vi "Lab1-my.vi"() -> ()   [LabVIEW 2013]
uses:
  <vilib>/Instr/_visa.llb/VISA Configure Serial Port (Instr).vi
panel:
  in  "file (use dialog)":path
  in  "stop everything":bool
  in  "send request":bool
  in  "Timeout [ms]":u32=5000
  out "answer":string
  in  "request":string
  in  "parity (0:none)":enum16{"None", "Odd", "Even", "Mark", "Space"}(ring)
  in  "data bits (8)":u16=8 min=5 max=8 step=1
  in  "baud rate (9600)":u32=9600
  in  "VISA resource name":refnum<visa-resource-name>
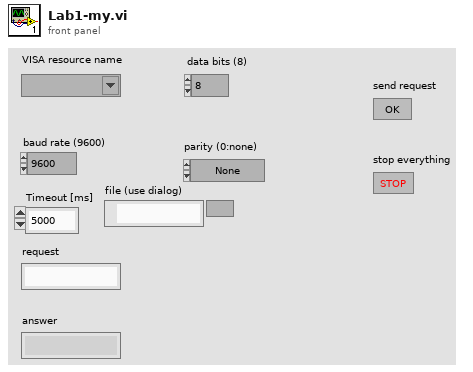
[diagram p1: front panel]
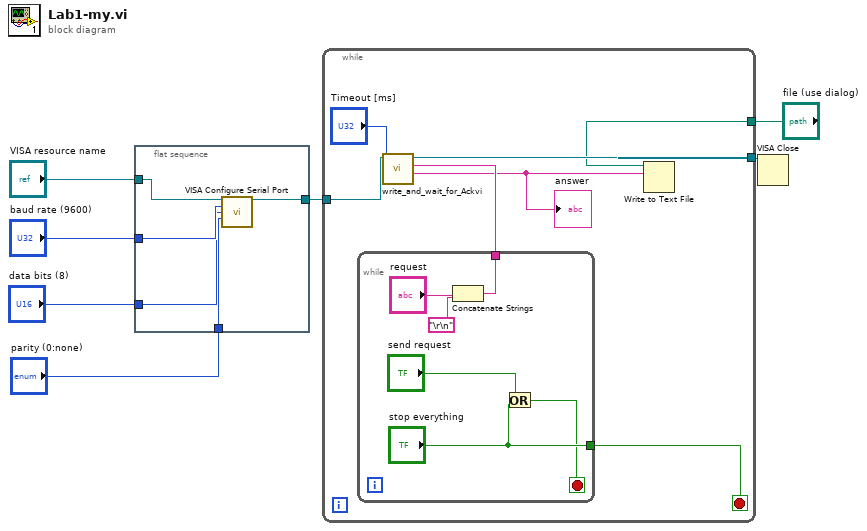
[diagram p0: block diagram]
diagram:
  n1 = flat-sequence {
    tunnel: "VISA resource name" -> [w12]
    tunnel: "baud rate (9600)" -> [w11]
    tunnel: "data bits (8)" -> [w10]
    tunnel: "parity (0:none)" -> [w9]
    tunnel: [w8] -> w3
    frame #0 {
      n2 = call-poly "VISA Configure Serial Port"("VISA resource name"=w12, "baud rate (9600)"=w11, "data bits (8)"=w10, "parity (0:none)"=w9) -> ("VISA resource name out"=w8:refnum<visa-resource-name>)  [unwired: 10 in, 1 out]
    }
  }
  n3 = while {
    tunnel: w3 -> [w19]
    tunnel: [w18] -> w2
    tunnel: "file (use dialog)" -> [w13]
    stop <- w15 stop-if-true
    n4 = while {
      tunnel: [w23] -> w17
      tunnel: ["stop everything"] -> w15
      stop <- w20 stop-if-true
      n5 = Concatenate Strings("request", "\r\n") -> (w23:string)
      n6 = Or(x="send request", y="stop everything") -> (x .or. y?=w20:bool)
    }
    n7 = call "write_and_wait_for_Ackvi.vi"("request"=w17, "Timeout [ms]"="Timeout [ms]", "VISA resource name"=w19) -> ("result"=w14:string, "VISA resource name out"=w18:refnum<visa-resource-name>)  [unwired: 4 in, 1 out]
    "answer" <- w14
    n8 = Write to Text File(file (use dialog)=w13, text=w14) -> ()  [unwired: 2 in, 3 out]
  }
  n9 = VISA Close(VISA resource name=w2) -> ()  [unwired: 1 in, 1 out]
